vi "save-monocoupSD.vi"(0 "Multiplie le nombre de spectres":i32=10, 1 "Ref":bool=TRUE, 2 "AbsTrans":bool=TRUE, 3 "BGR":bool, 4 "BGS":bool, 5 "Sig":bool=TRUE, 6 "Digital in":refnum<vi>) -> ()   [LabVIEW 2015]
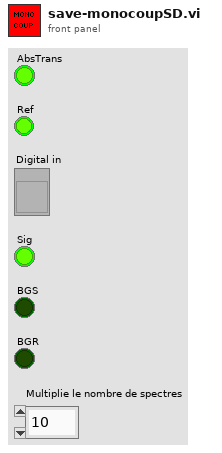
[diagram p1: front panel]
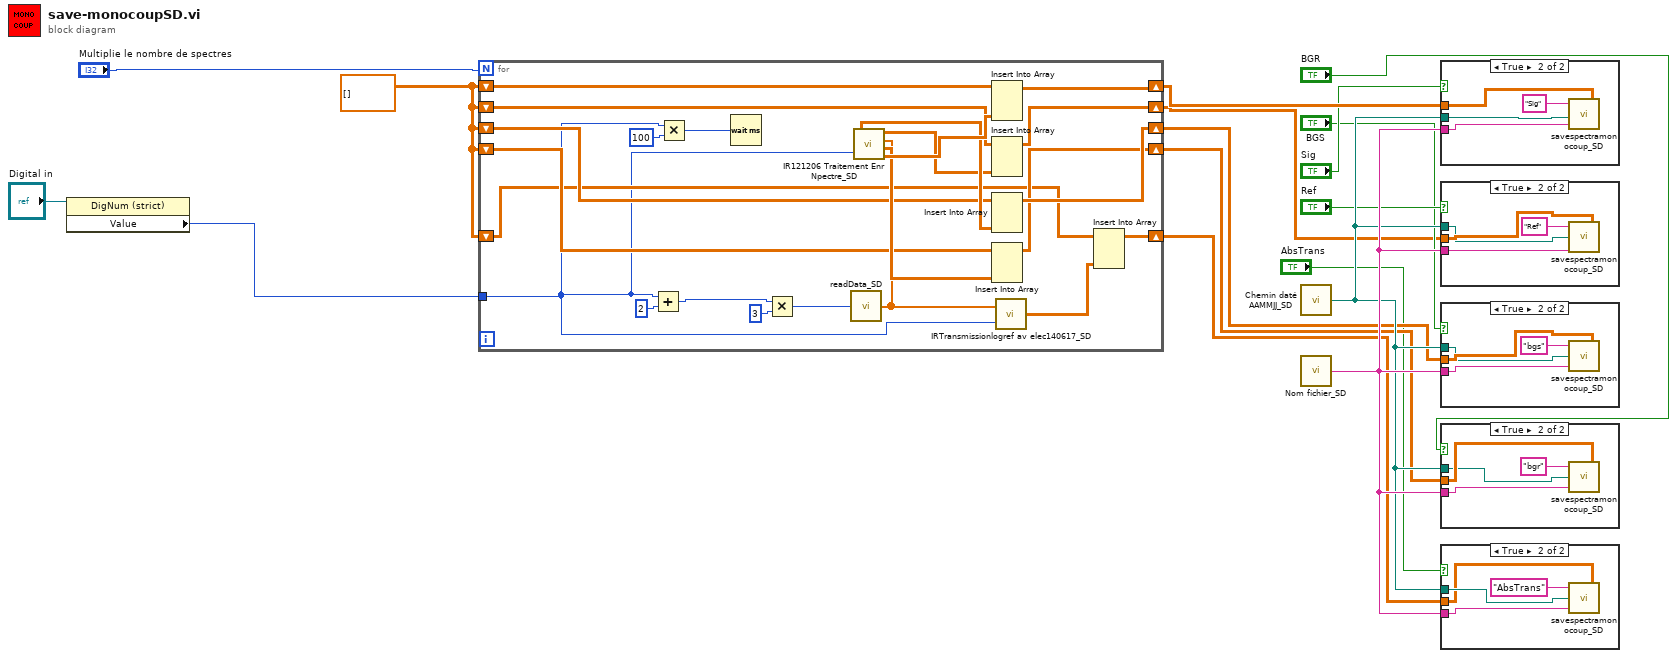
[diagram p0: block diagram]
diagram:
  w4 = dbl[][] [] ("SIg-Bg")
  n1 = property class="DigNum (strict)"(reference="Digital in") -> ("Value"=w16:i32)  [unwired: 1 in, 2 out]
  n2 = for {
    N: "Multiplie le nombre de spectres" -> [_]
    tunnel: w16 -> [w20]
    shift-right: [w28] -> w14
    shift-left: w4 -> [w32]
    shift-right: [w26] -> w6
    shift-left: w4 -> [w30]
    shift-right: [w27] -> w7
    shift-left: w4 -> [w31]
    shift-right: [w25] -> w5
    shift-left: w4 -> [w29]
    shift-right: [w24] -> w3
    shift-left: w4 -> [w23]
    n3 = Add(x=w20, y=2) -> (x+y=w37:i32)
    n4 = Multiply(x=w20, y=100) -> (x*y=w21:i32)
    n5 = Wait (ms)(milliseconds to wait=w21) -> ()  [unwired: 1 out]
    n6 = Multiply(x=w37, y=3) -> (x*y=w18:i32)
    n7 = call "readData_SD.vi"("how many points"=w18) -> ("résultat début série"=w17:dbl[])
    n8 = call "IR121206 Traitement Enr Npectre_SD.vi"("Moyenne par pas"=w20, "resultat_input"=w17) -> ("BgSig"=w34:dbl[][], "Ref-Bg"=w33:dbl[][], "BgRef"=w35:dbl[][], "Sig-Bg"=w36:dbl[][])
    n9 = Insert Into Array(array=w32, new element=w36) -> (w28:dbl[][])  [unwired: 2 in]
    n10 = Insert Into Array(array=w31, new element=w33) -> (w27:dbl[][])  [unwired: 2 in]
    n11 = Insert Into Array(array=w30, new element=w34) -> (w26:dbl[][])  [unwired: 2 in]
    n12 = Insert Into Array(array=w29, new element=w35) -> (w25:dbl[][])  [unwired: 2 in]
    n13 = call "IRTransmissionlogref av elec140617_SD.vi"("Moyenne par pas"=w20, "resultat_input"=w17) -> ("Résultat DO"=w19:dbl[][])
    n14 = Insert Into Array(array=w23, new element=w19) -> (w24:dbl[][])  [unwired: 2 in]
  }
  n15 = call "Chemin daté AAMMJJ_SD.vi"() -> ("chemin du dossier"=w13:path)
  n16 = call "Nom fichier_SD.vi"() -> ("nom"=w15:string)
  n17 = case shown="True" "Sig" {
    tunnel: w13 -> [_ w42]
    tunnel: w14 -> [_ w41]
    tunnel: w15 -> [_ w40]
    frame False {
    }
    frame True {
      n18 = call "savespectramonocoup_SD.vi"("Data"=w41, "nom"=w40, "chemin du dossier"=w42, "String"="Sig") -> ()
    }
  }
  n19 = case shown="True" "Ref" {
    tunnel: w13 -> [_ w44]
    tunnel: w15 -> [_ w47]
    tunnel: w7 -> [_ w45]
    frame False {
    }
    frame True {
      n20 = call "savespectramonocoup_SD.vi"("Data"=w45, "nom"=w47, "chemin du dossier"=w44, "String"="Ref") -> ()
    }
  }
  n21 = case shown="True" "BGS" {
    tunnel: w13 -> [_ w48]
    tunnel: w15 -> [_ w50]
    tunnel: w6 -> [_ w49]
    frame False {
    }
    frame True {
      n22 = call "savespectramonocoup_SD.vi"("Data"=w49, "nom"=w50, "chemin du dossier"=w48, "String"="bgs") -> ()
    }
  }
  n23 = case shown="True" "BGR" {
    tunnel: w13 -> [_ w53]
    tunnel: w15 -> [_ w52]
    tunnel: w5 -> [_ w55]
    frame False {
    }
    frame True {
      n24 = call "savespectramonocoup_SD.vi"("Data"=w55, "nom"=w52, "chemin du dossier"=w53, "String"="bgr") -> ()
    }
  }
  n25 = case shown="True" "AbsTrans" {
    tunnel: w13 -> [_ w57]
    tunnel: w15 -> [_ w58]
    tunnel: w3 -> [_ w56]
    frame False {
    }
    frame True {
      n26 = call "savespectramonocoup_SD.vi"("Data"=w56, "nom"=w58, "chemin du dossier"=w57, "String"="AbsTrans") -> ()
    }
  }
